vi "intensity_calibration_old.vi"(6 "appended path":path, 8 "Boolean":bool, 9 "array in":u16[][](array[numeric]), 10 "Value":T1={"Packet Size"=1500, "Pixel Format"=17825797, "Gain in dB"=1.0, "Exposure Time in µs"=1500, "Stream Bytes per Second"=50000000} caption="Control Camera Properties" {"Stream Bytes per Second" min=1000000 max=124000000 step=100000 format="%.1p"; "Exposure Time in µs" min=21 max=153391689 format="%#.0f"; "Gain in dB" min=0.0 max=26.0 format="%#_2g"; "Pixel Format" items=["Mono 12 Packed"=17563654, "Mono 12"=17825797]}, 11 "reference":refnum<vi>) -> (1 "array out":u16[][](array[numeric]))   [LabVIEW 2014]
uses:
  type definitions/control camera properties.ctl
  <vilib>/Utility/file.llb/Read From Spreadsheet File (DBL).vi
panel:
  out "interpolated data":dbl[][](array[numeric])
  out "min value":dbl
  out "max value":dbl
  # "Bytes"
  # "Trigger"
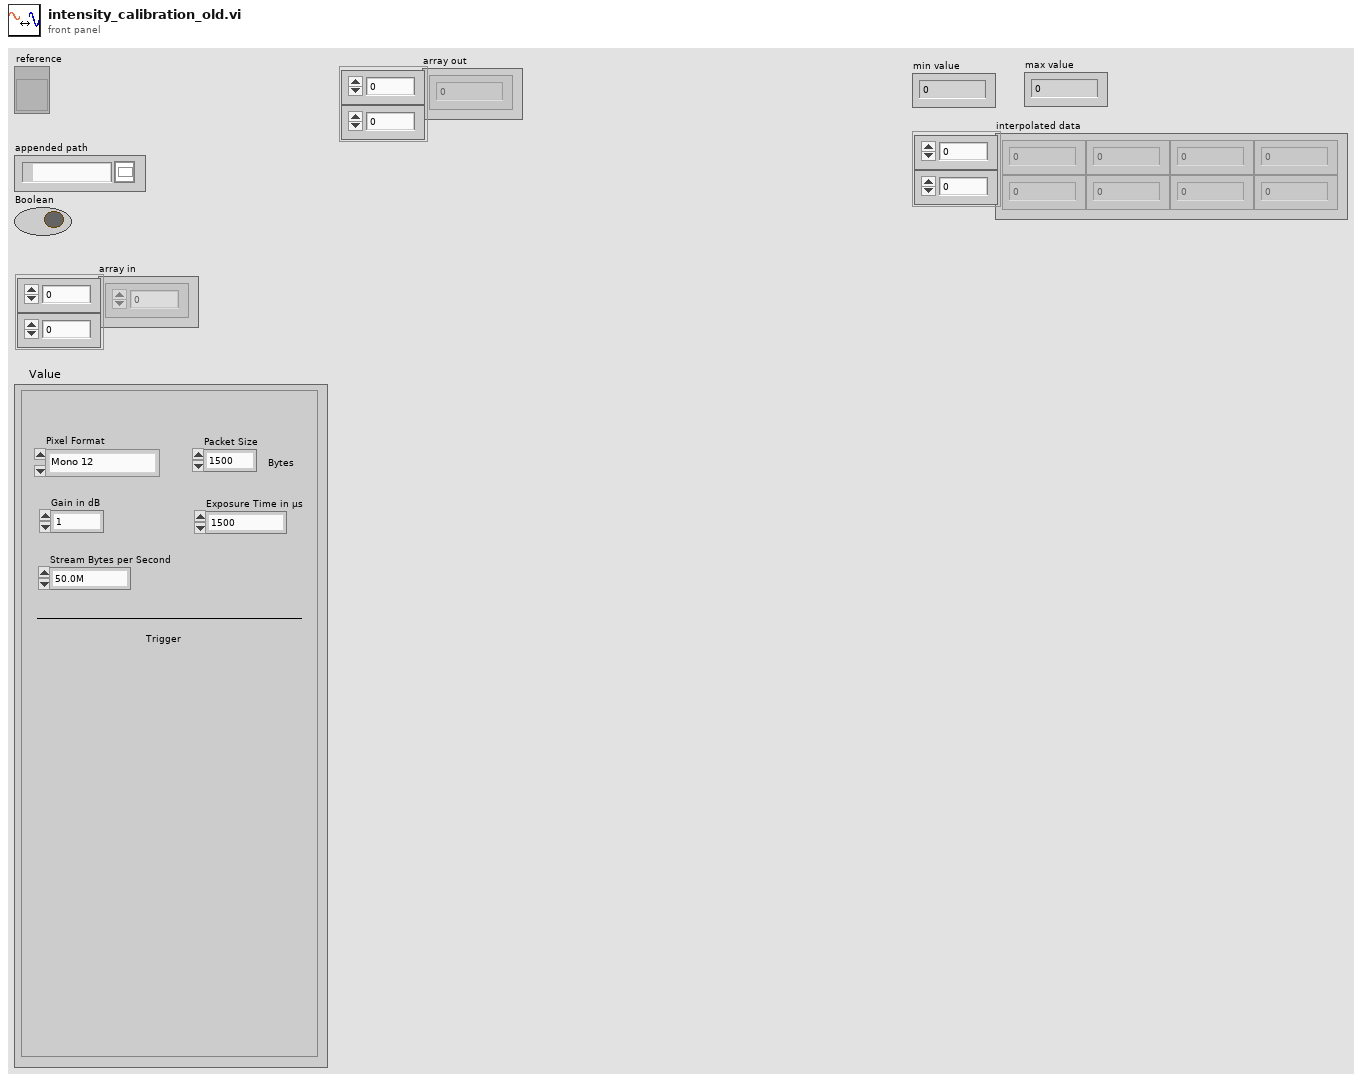
[diagram p1: front panel]
types:
  T1 = typedef "control camera properties.ctl" = cluster{"Packet Size":u32, "Pixel Format":u32, "Gain in dB":dbl, "Exposure Time in µs":u32, "Stream Bytes per Second":u32}
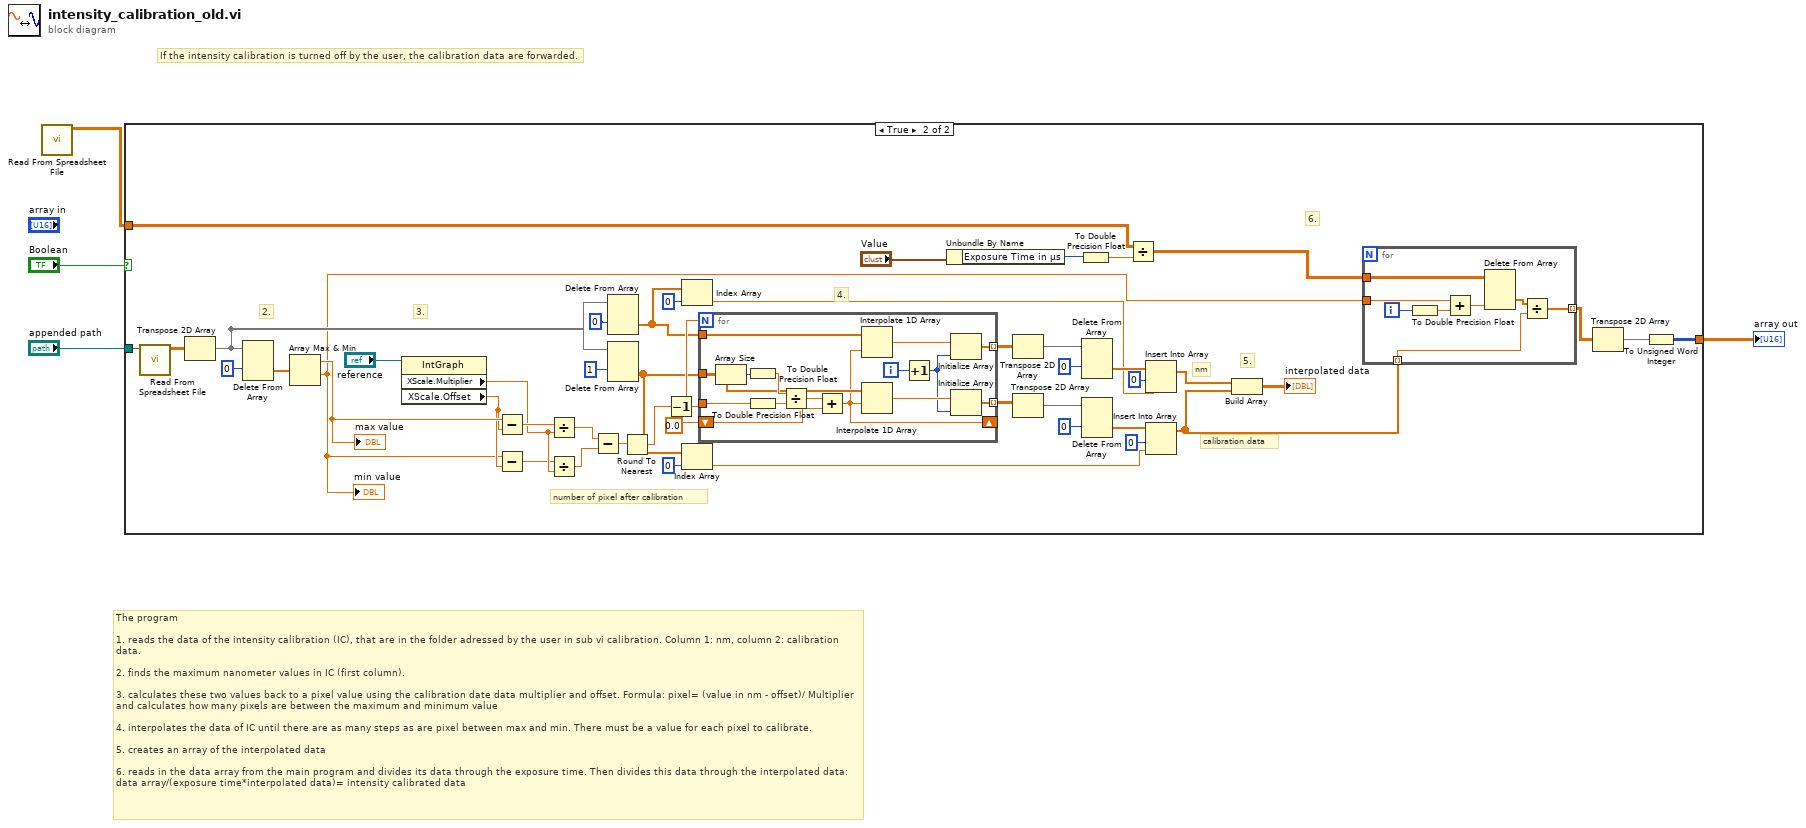
[diagram p0: block diagram]
diagram:
  # "If the intensity calibration is turned off by the user, the calibration data are forwarded."
  # "The program\n\n1. reads the data of the intensity calibration (IC), that are in the folder adressed by the user in sub vi calibration. Column 1: nm, column 2: calibration data.\n\n2. finds the maximum nanometer values in IC (first column). \n\n3. calculates these two values back to a pixel value using the calibration date data multiplier and offset. Formula: pixel= (value in nm - offset)/ Multiplier\nand calculates how many pixels are between the maximum and minimum value\n\n4. interpolates the data of IC until there are as many steps as are pixel between max and min. There must be a value for each pixel to calibrate.\n\n5. creates an array of the interpolated data\n\n6. reads in the data array from the main program and divides its data through the exposure time. Then divides this data through the interpolated data:\ndata array/(exposure time*interpolated data)= intensity calibrated data"
  n1 = call-poly <vilib>:"Read From Spreadsheet File.vi"() -> ("all rows"=w1:dbl[][])  [unwired: 7 in, 4 out]
  n2 = case shown="True" "Boolean" {
    tunnel: "appended path" -> [_ w52]
    tunnel: [w5 w7] -> w2
    tunnel: w1 -> [w5 w6]
    frame False {
    }
    frame True {
      # "6."
      # "5."
      # "4."
      # "3."
      # "2."
      # "calibration data"
      # "nm"
      # "number of pixel after calibration"
      n3 = call-poly <vilib>:"Read From Spreadsheet File.vi"("file path (dialog if empty)"=w52) -> ("all rows"=w49:dbl[][])  [unwired: 6 in, 4 out]
      n4 = Transpose 2D Array(2D array=w49) -> (transposed array=w18:dbl[][])
      n5 = Delete From Array(array=w18, index (row)=0) -> (deleted portion=w50:dbl[])  [unwired: 2 in, 1 out]
      n6 = Array Max & Min(array=w50) -> (max value=w47:dbl, min value=w9:dbl)  [unwired: 2 out]
      "max value" <- w47
      "min value" <- w9
      n7 = property on="Property Node" class="IntGraph"(reference="reference") -> ("XScale.Multiplier"=w44:dbl, "XScale.Offset"=w46:dbl)  [unwired: 1 in, 2 out]
      n8 = Subtract(x=w47, y=w46) -> (x-y=w45:dbl)
      n9 = Subtract(x=w9, y=w46) -> (x-y=w43:dbl)
      n10 = Divide(x=w45, y=w44) -> (x/y=w41:dbl)
      n11 = Divide(x=w43, y=w44) -> (x/y=w42:dbl)
      n12 = Subtract(x=w41, y=w42) -> (x-y=w40:dbl)
      n13 = Delete From Array(array=w18, index (row)=0 ("length")) -> (deleted portion=w29:dbl[])  [unwired: 2 in, 1 out]
      n14 = Delete From Array(array=w18, index (row)=1) -> (deleted portion=w26:dbl[])  [unwired: 2 in, 1 out]
      n15 = Round To Nearest(number=w40) -> (nearest integer value=w19:dbl)
      n16 = Decrement(x=w19) -> (x-1=w36:dbl)
      n17 = Index Array(array=w29, index=0) -> (element=w24:dbl)
      n18 = Index Array(array=w26, index=0) -> (element=w20:dbl)
      n19 = for {
        N: w36 -> [_]
        tunnel: w26 -> [w64]
        tunnel: w36 -> [w67]
        tunnel: [w73] -> w37 mode=indexing
        shift-right: [w62] -> _
        shift-left: 0.0 -> [w71]
        tunnel: [w65] -> w31 mode=indexing
        tunnel: w29 -> [w63]
        i -> [w74]
        n20 = Array Size(array=w64) -> (size(s)=w69:i32)
        n21 = To Double Precision Float(number=w69) -> (double precision float=w70:dbl)
        n22 = To Double Precision Float(number=w67) -> (double precision float=w68:dbl)
        n23 = Divide(x=w70, y=w68) -> (x/y=w72:dbl)
        n24 = Add(x=w72, y=w71) -> (x+y=w62:dbl)
        n25 = Interpolate 1D Array(1:w62, 2:w63) -> (0:w61:dbl)
        n26 = Interpolate 1D Array(1:w62, 2:w64) -> (0:w75:dbl)
        n27 = Increment(x=w74) -> (x+1=w66:i32)
        n28 = Initialize Array(w61, w66) -> (w65:dbl[])
        n29 = Initialize Array(w75, w66) -> (w73:dbl[])
      }
      n30 = Unbundle By Name("Value") -> ("Exposure Time in µs"=w10:u32)
      n31 = Transpose 2D Array(2D array=w31) -> (transposed array=w30:dbl[][])
      n32 = Transpose 2D Array(2D array=w37) -> (transposed array=w34:dbl[][])
      n33 = To Double Precision Float(number=w10) -> (double precision float=w11:dbl)
      n34 = Delete From Array(array=w30, index (row)=0) -> (deleted portion=w25:dbl[])  [unwired: 2 in, 1 out]
      n35 = Delete From Array(array=w34, index (row)=0) -> (deleted portion=w21:dbl[])  [unwired: 2 in, 1 out]
      n36 = Divide(x=w6, y=w11) -> (x/y=w13:dbl[][])
      n37 = Insert Into Array(array=w25, index=0, new element=w24) -> (w16:dbl[])
      n38 = Insert Into Array(array=w21, index=0, new element=w20) -> (w15:dbl[])
      n39 = Build Array(w16, w15) -> (→"interpolated data":dbl[][])
      n40 = for {
        tunnel: w13 -> [w60]
        tunnel: w15 -> [w57] mode=indexing
        tunnel: [w58] -> w14 mode=indexing
        tunnel: w9 -> [w56]
        i -> [w54]
        n41 = To Double Precision Float(number=w54) -> (double precision float=w53:dbl)
        n42 = Add(x=w56, y=w53) -> (x+y=w55:dbl)
        n43 = Delete From Array(array=w60, index (col)=w55) -> (deleted portion=w59:dbl[])  [unwired: 2 in, 1 out]
        n44 = Divide(x=w59, y=w57) -> (x/y=w58:dbl[])
      }
      n45 = Transpose 2D Array(2D array=w14) -> (transposed array=w8:dbl[][])
      n46 = To Unsigned Word Integer(number=w8) -> (unsigned 16bit integer=w7:u16[][])
    }
  }
  "array out" <- w2
